vi "DROPBEAR_Model_Updating_Initialize.vi"(8 "error in (no error)":errorcluster, 11 "DROPBEAR_Model_Updating in":refnum<class "DROPBEAR_Model_Updating.lvclass">) -> (0 "error out":errorcluster, 3 "DROPBEAR_Model_Updating out":refnum<class "DROPBEAR_Model_Updating.lvclass">)   [LabVIEW 2021, in "DROPBEAR_Model_Updating.lvclass"]
uses:
  DROPBEAR_Model_Updating.lvclass
  DROPBEAR_Model_Updating.lvclass/DROPBEAR_Model_Updating.ctl
  MOCKBEAR/MOCKBEAR.lvclass
  FEA_Model/FEA_Model.lvclass
  Data_Array/Data_Array.lvclass
  Moving_Statistic/Moving_Statistic.lvclass
  Online_Statistic/Online_Statistic.lvclass
  Kalman_Filter/Kalman_Filter.lvclass
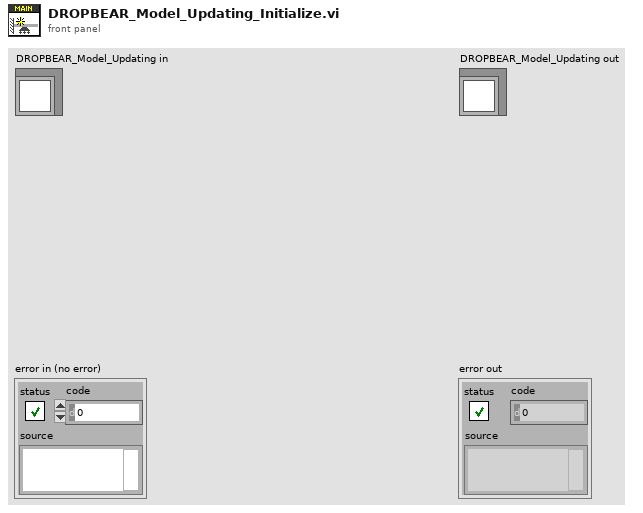
[diagram p1: front panel]
types:
  T1 = cluster{"Measurement Variance":dbl, "State Variance":dbl, "Threshold":dbl}
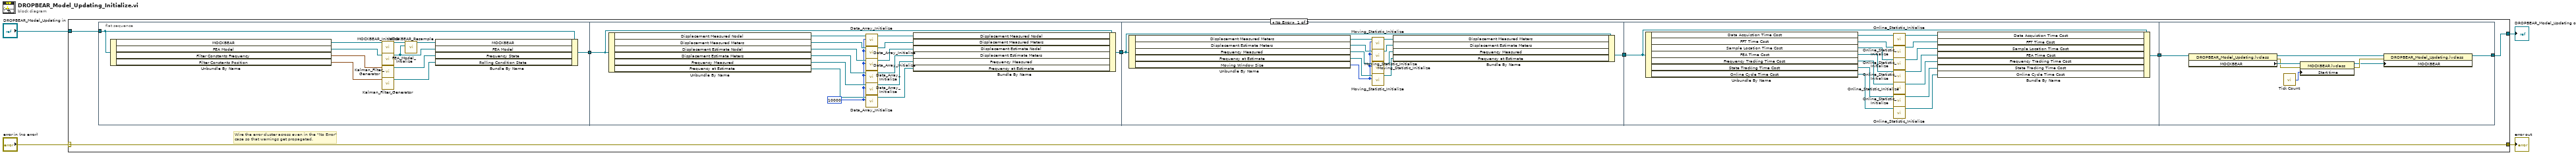
[diagram p0: block diagram]
diagram:
  n1 = case shown="No Error" "error in (no error)" {
    selector: "error in (no error)" -> [w11 w74]
    tunnel: [w11 w74] -> w3
    tunnel: [w6 w73] -> w1
    tunnel: "DROPBEAR_Model_Updating in" -> [w7 w73]
    frame No Error {
      # "Wire the error cluster across even in the \"No Error\"\ncase so that warnings get propagated."
      n2 = flat-sequence {
        tunnel: w7 -> [w16]
        tunnel: [w17] -> w10
        tunnel: w10 -> [w31]
        tunnel: [w24] -> w9
        tunnel: w9 -> [w43]
        tunnel: [w38] -> w8
        tunnel: w8 -> [w57]
        tunnel: [w49] -> w5
        tunnel: [w65] -> w6
        tunnel: w5 -> [w72]
        frame #0 {
          n3 = Unbundle By Name(w16) -> ("MOCKBEAR"=w21:refnum<class "MOCKBEAR.lvclass">, "FEA Model"=w22:refnum<class "FEA_Model.lvclass">, "Filter Constants Frequency"=w13:T1, "Filter Constants Position"=w12:T1)
          n4 = call-dynamic "MOCKBEAR_Initialize.vi"("MOCKBEAR in"=w21) -> ("MOCKBEAR out"=w20:refnum<class "MOCKBEAR.lvclass">)  [unwired: 9 in, 1 out]
          n5 = call-dynamic "FEA_Model_Intialize.vi"("FEA_Model in"=w22) -> ("FEA_Model out"=w18:refnum<class "FEA_Model.lvclass">)  [unwired: 9 in, 1 out]
          n6 = call "Kalman_Filter_Generator.vi"("Filter Constants"=w13) -> ("Kalman_Filter out"=w15:refnum<class "Kalman_Filter.lvclass">)  [unwired: 9 in, 1 out]
          n7 = call "Kalman_Filter_Generator.vi"("Filter Constants"=w12) -> ("Kalman_Filter out"=w14:refnum<class "Kalman_Filter.lvclass">)  [unwired: 9 in, 1 out]
          n8 = call-dynamic "MOCKBEAR_Resample.vi"("FEA_Model in"=w18, "MOCKBEAR in"=w20) -> ("MOCKBEAR out"=w19:refnum<class "MOCKBEAR.lvclass">)  [unwired: 8 in, 1 out]
          n9 = Bundle By Name(cluster=w16, "MOCKBEAR"=w19, "FEA Model"=w18, "Frequency State"=w15, "Rolling Condition State"=w14) -> (w17:refnum<class "DROPBEAR_Model_Updating.lvclass">)
        }
        frame #1 {
          w23 = 10000
          n10 = Unbundle By Name(w31) -> ("Displacement Measured Nodal"=w37:refnum<class "Data_Array.lvclass">, "Displacement Measured Meters"=w36:refnum<class "Data_Array.lvclass">, "Displacement Estimate Nodal"=w35:refnum<class "Data_Array.lvclass">, "Displacement Estimate Meters"=w34:refnum<class "Data_Array.lvclass">, "Frequency Measured"=w33:refnum<class "Data_Array.lvclass">, "Frequency at Estimate"=w32:refnum<class "Data_Array.lvclass">)
          n11 = call-dynamic "Data_Array_Initialize.vi"("Buffer"=w23, "Data_Array in"=w37) -> ("Data_Array out"=w30:refnum<class "Data_Array.lvclass">)  [unwired: 8 in, 1 out]
          n12 = call-dynamic "Data_Array_Initialize.vi"("Buffer"=w23, "Data_Array in"=w36) -> ("Data_Array out"=w29:refnum<class "Data_Array.lvclass">)  [unwired: 8 in, 1 out]
          n13 = call-dynamic "Data_Array_Initialize.vi"("Buffer"=w23, "Data_Array in"=w35) -> ("Data_Array out"=w28:refnum<class "Data_Array.lvclass">)  [unwired: 8 in, 1 out]
          n14 = call-dynamic "Data_Array_Initialize.vi"("Buffer"=w23, "Data_Array in"=w34) -> ("Data_Array out"=w27:refnum<class "Data_Array.lvclass">)  [unwired: 8 in, 1 out]
          n15 = call-dynamic "Data_Array_Initialize.vi"("Buffer"=w23, "Data_Array in"=w33) -> ("Data_Array out"=w26:refnum<class "Data_Array.lvclass">)  [unwired: 8 in, 1 out]
          n16 = call-dynamic "Data_Array_Initialize.vi"("Buffer"=w23, "Data_Array in"=w32) -> ("Data_Array out"=w25:refnum<class "Data_Array.lvclass">)  [unwired: 8 in, 1 out]
          n17 = Bundle By Name(cluster=w31, "Displacement Measured Nodal"=w30, "Displacement Measured Meters"=w29, "Displacement Estimate Nodal"=w28, "Displacement Estimate Meters"=w27, "Frequency Measured"=w26, "Frequency at Estimate"=w25) -> (w24:refnum<class "DROPBEAR_Model_Updating.lvclass">)
        }
        frame #2 {
          n18 = Unbundle By Name(w43) -> ("Displacement Measured Meters"=w48:refnum<class "Moving_Statistic.lvclass">, "Displacement Estimate Meters"=w47:refnum<class "Moving_Statistic.lvclass">, "Frequency Measured"=w46:refnum<class "Moving_Statistic.lvclass">, "Frequency at Estimate"=w45:refnum<class "Moving_Statistic.lvclass">, "Moving Window Size"=w44:i32)
          n19 = call-dynamic "Moving_Statistic_Initialize.vi"("Window"=w44, "Moving_Mean in"=w48) -> ("Moving_Mean out"=w42:refnum<class "Moving_Statistic.lvclass">)  [unwired: 8 in, 1 out]
          n20 = call-dynamic "Moving_Statistic_Initialize.vi"("Window"=w44, "Moving_Mean in"=w47) -> ("Moving_Mean out"=w41:refnum<class "Moving_Statistic.lvclass">)  [unwired: 8 in, 1 out]
          n21 = call-dynamic "Moving_Statistic_Initialize.vi"("Window"=w44, "Moving_Mean in"=w46) -> ("Moving_Mean out"=w40:refnum<class "Moving_Statistic.lvclass">)  [unwired: 8 in, 1 out]
          n22 = call-dynamic "Moving_Statistic_Initialize.vi"("Window"=w44, "Moving_Mean in"=w45) -> ("Moving_Mean out"=w39:refnum<class "Moving_Statistic.lvclass">)  [unwired: 8 in, 1 out]
          n23 = Bundle By Name(cluster=w43, "Displacement Measured Meters"=w42, "Displacement Estimate Meters"=w41, "Frequency Measured"=w40, "Frequency at Estimate"=w39) -> (w38:refnum<class "DROPBEAR_Model_Updating.lvclass">)
        }
        frame #3 {
          n24 = Unbundle By Name(w57) -> ("Data Acquistion Time Cost"=w64:refnum<class "Online_Statistic.lvclass">, "FFT Time Cost"=w63:refnum<class "Online_Statistic.lvclass">, "Sample Location Time Cost"=w62:refnum<class "Online_Statistic.lvclass">, "FEA Time Cost"=w61:refnum<class "Online_Statistic.lvclass">, "Frequency Tracking Time Cost"=w60:refnum<class "Online_Statistic.lvclass">, "State Tracking Time Cost"=w59:refnum<class "Online_Statistic.lvclass">, "Online Cycle Time Cost"=w58:refnum<class "Online_Statistic.lvclass">)
          n25 = call-dynamic "Online_Statistic_Initialize.vi"("Online_Statistic in"=w64) -> ("Online_Statistic out"=w56:refnum<class "Online_Statistic.lvclass">)  [unwired: 9 in, 1 out]
          n26 = call-dynamic "Online_Statistic_Initialize.vi"("Online_Statistic in"=w63) -> ("Online_Statistic out"=w55:refnum<class "Online_Statistic.lvclass">)  [unwired: 9 in, 1 out]
          n27 = call-dynamic "Online_Statistic_Initialize.vi"("Online_Statistic in"=w62) -> ("Online_Statistic out"=w54:refnum<class "Online_Statistic.lvclass">)  [unwired: 9 in, 1 out]
          n28 = call-dynamic "Online_Statistic_Initialize.vi"("Online_Statistic in"=w61) -> ("Online_Statistic out"=w53:refnum<class "Online_Statistic.lvclass">)  [unwired: 9 in, 1 out]
          n29 = call-dynamic "Online_Statistic_Initialize.vi"("Online_Statistic in"=w60) -> ("Online_Statistic out"=w52:refnum<class "Online_Statistic.lvclass">)  [unwired: 9 in, 1 out]
          n30 = call-dynamic "Online_Statistic_Initialize.vi"("Online_Statistic in"=w59) -> ("Online_Statistic out"=w51:refnum<class "Online_Statistic.lvclass">)  [unwired: 9 in, 1 out]
          n31 = call-dynamic "Online_Statistic_Initialize.vi"("Online_Statistic in"=w58) -> ("Online_Statistic out"=w50:refnum<class "Online_Statistic.lvclass">)  [unwired: 9 in, 1 out]
          n32 = Bundle By Name(cluster=w57, "Data Acquistion Time Cost"=w56, "FFT Time Cost"=w55, "Sample Location Time Cost"=w54, "FEA Time Cost"=w53, "Frequency Tracking Time Cost"=w52, "State Tracking Time Cost"=w51, "Online Cycle Time Cost"=w50) -> (w49:refnum<class "DROPBEAR_Model_Updating.lvclass">)
        }
        frame #4 {
          n33 = property class="DROPBEAR_Model_Updating.lvclass"(reference=w72) -> (reference out=w66:refnum<class "DROPBEAR_Model_Updating.lvclass">, error out=w69:errorcluster, "MOCKBEAR"=w71:refnum<class "MOCKBEAR.lvclass">)  [unwired: 1 in]
          n34 = call "Tick Count"() -> ("Tick Count(uSec)"=w70:u32)
          n35 = property class="MOCKBEAR.lvclass"(reference=w71, error in=w69, "Start time"=w70) -> (reference out=w67:refnum<class "MOCKBEAR.lvclass">, error out=w68:errorcluster)
          n36 = property class="DROPBEAR_Model_Updating.lvclass"(reference=w66, error in=w68, "MOCKBEAR"=w67) -> (reference out=w65:refnum<class "DROPBEAR_Model_Updating.lvclass">)  [unwired: 1 out]
        }
      }
    }
    frame Error {
    }
  }
  "error out" <- w3
  "DROPBEAR_Model_Updating out" <- w1
